vi "Host vi.vi"() -> ()   [LabVIEW 2017]
uses:
  <vilib>/FPGAPlugInAG/USB-7856R/niLvFpga_Open_USB-7856R.vi
  <vilib>/rvi/interface/common/dynamic/niFpgaDynamicAddResources.vi
  <vilib>/Utility/error.llb/Error Cluster From Error Code.vi
  <vilib>/rvi/errors/niLvFpgaAdjustHostInterfaceError.vi
  <vilib>/FPGAPlugInAG/Dynamic/niLvFpga_Close_Dynamic.vi
  <vilib>/rvi/interface/nirviOpenFPGA/nirviOpenFPGA.xnode
  FPGA Bitfiles/FIFOtest_FPGATarget_FPGA_UHdwu-gc-TM.lvbitx
  FPGA.vi
  <vilib>/rvi/interface/nirviMethod/nirviMethod.xnode
  <vilib>/rvi/interface/nirviReadWriteControl/nirviReadWriteControl.xnode
  <vilib>/rvi/interface/nirviCloseFPGA/nirviCloseFPGA.xnode
  NiFpgaLv.dll
  <vilib>/rvi/interface/Simulation/niFpgaSimulationCallBeginRW.vi
  <vilib>/FPGAPlugInAG/Dynamic/niLvFpga_ReadFifo_Dynamic.vi
  <vilib>/rvi/errors/niLvFpgaMergeErrorWithErrorCode.vi
panel:
  out "Data":u16[](array[numeric])
  out "Loop counter 2":i32
  out "Loop counter 1":i32
  in  "stop":bool
  in  "Nmax":i32=5
  in  "Pop\nhost FIFO":bool
  out "Elements Remaining":u32
  out "Number of Elements to Write":u32=1023
  in  "Push\ntarget FIFO":bool
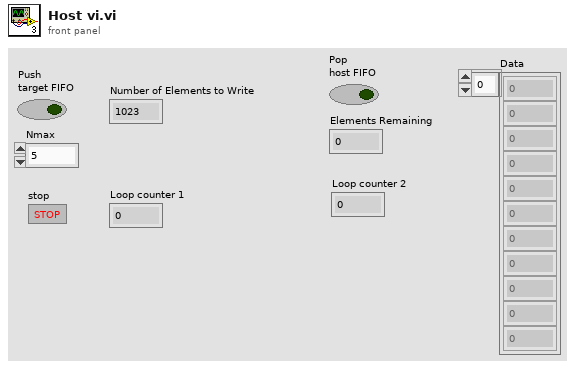
[diagram p1: front panel]
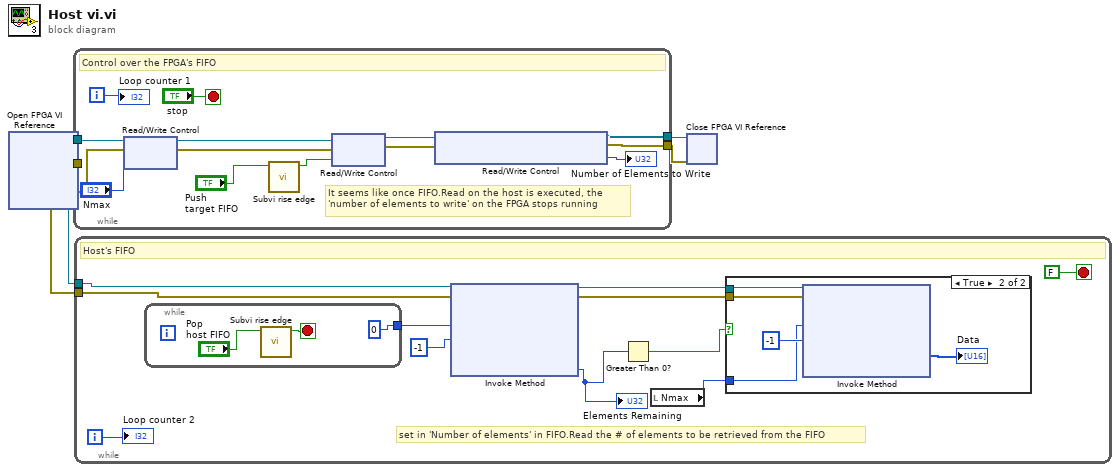
[diagram p0: block diagram]
diagram:
  n1 = xnode "Open FPGA VI Reference"() -> ("FPGA VI Reference Out"=w1:refnum<k20>, "error out"=w2:errorcluster)  [unwired: 2 in]
  n2 = while {
    tunnel: w1 -> [w16]
    tunnel: w2 -> [w14]
    tunnel: [w18] -> w4
    tunnel: [w17] -> w3
    i -> [w11]
    stop <- "stop" stop-if-true
    # "It seems like once FIFO.Read on the host is executed, the\n'number of elements to write' on the FPGA stops running"
    # "Control over the FPGA's FIFO"
    n3 = xnode "Read/Write Control"("FPGA VI Reference In"=w16, "error in"=w14, "Nmax"="Nmax") -> ("FPGA VI Reference Out"=w15:refnum<k20>, "error out"=w13:errorcluster)
    n4 = call "Subvi rise edge.vi"("Start"="Push\ntarget FIFO") -> ("Boolean"=w6:bool)  [unwired: 10 in]
    n5 = xnode "Read/Write Control"("FPGA VI Reference In"=w15, "error in"=w13, "Start"=w6) -> ("FPGA VI Reference Out"=w10:refnum<k20>, "error out"=w9:errorcluster)
    n6 = xnode "Read/Write Control"("FPGA VI Reference In"=w10, "error in"=w9) -> ("FPGA VI Reference Out"=w18:refnum<k20>, "error out"=w17:errorcluster, "Number of Elements to Write"=→"Number of Elements to Write":u32)
    "Loop counter 1" <- w11
  }
  n7 = while {
    tunnel: w1 -> [w29]
    tunnel: w2 -> [w28]
    i -> [w26]
    stop <- FALSE stop-if-true
    # "set in 'Number of elements' in FIFO.Read the # of elements to be retrieved from the FIFO"
    # "Host's FIFO"
    n8 = while {
      tunnel: [u32 0 ("Number of Elements")] -> w19
      stop <- w36 stop-if-true
      n9 = call "Subvi rise edge.vi"("Start"="Pop\nhost FIFO") -> ("Boolean"=w36:bool)  [unwired: 10 in]
    }
    n10 = xnode "Invoke Method"("FPGA VI Reference In"=w29, "error in"=w28, "Number of Elements"=w19, "Timeout (ms)"=-1) -> ("FPGA VI Reference Out"=w24:refnum<k20>, "error out"=w23:errorcluster, "Elements Remaining"=w21:u32)  [unwired: 1 out]
    "Elements Remaining" <- w21
    n11 = Greater Than 0?(x=w21) -> (x > 0?=w20:bool)
    n12 = local read "Nmax"() -> (w22:i32)
    n13 = case shown="True" w20 {
      tunnel: w24 -> [_ w34]
      tunnel: w23 -> [_ w33]
      tunnel: w22 -> [_ w30]
      frame False {
      }
      frame True {
        n14 = xnode "Invoke Method"("FPGA VI Reference In"=w34, "error in"=w33, "Number of Elements"=w30, "Timeout (ms)"=-1) -> ("Data"=→"Data":u16[])  [unwired: 3 out]
      }
    }
    "Loop counter 2" <- w26
  }
  n15 = xnode "Close FPGA VI Reference"("FPGA VI Reference In"=w4, "error in"=w3) -> ()  [unwired: 1 out]
